vi "UnitTimestamp.vi"(8 "error in (no error)":errorcluster caption="错误输入（无错误）") -> (0 "error out":errorcluster caption="错误输出", 3 "字符串":string)   [LabVIEW 2018]
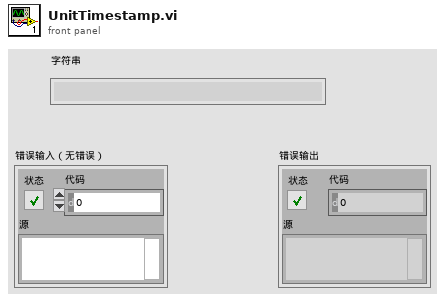
[diagram p1: front panel]
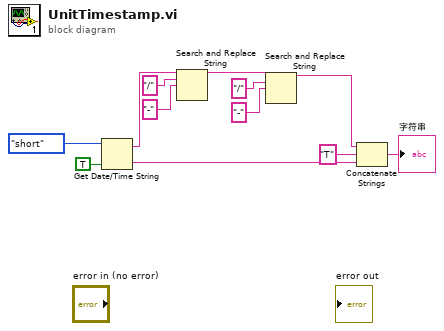
[diagram p0: block diagram]
diagram:
  n1 = Get Date/Time String(date format (0)=enum16{"short", "long", "abbreviated"}."short" ("日期格式(0)"), want seconds? (F)=TRUE ("需要秒？(F)")) -> (date string=w7:string, time string=w8:string)  [unwired: 1 in]
  n2 = Search and Replace String(input string=w7, search string="/" ("搜索字符串"), replace string="-" ("替换字符串(\"\")")) -> (result string=w2:string)  [unwired: 5 in, 3 out]
  n3 = Search and Replace String(input string=w2, search string="/" ("搜索字符串"), replace string="-" ("替换字符串(\"\")")) -> (result string=w1:string)  [unwired: 5 in, 3 out]
  n4 = Concatenate Strings(w1, "T", w8) -> (→"字符串":string)
